vi "Old Files Handler.vi"(8 "Error In":errorcluster, 11 "TDMS Log":refnum<class "TDMS Logger.lvclass">) -> (0 "Error Out":errorcluster, 3 "TDMS Log":refnum<class "TDMS Logger.lvclass">)   [LabVIEW 2015, in "TDMS Logger.lvlib" / "TDMS Logger.lvclass"]
uses:
  TDMS Logger.lvclass
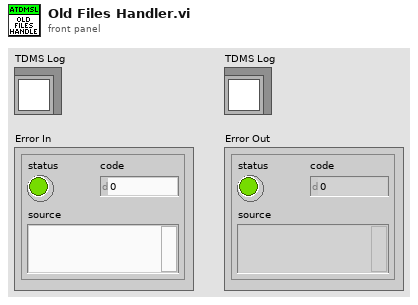
[diagram p1: front panel]
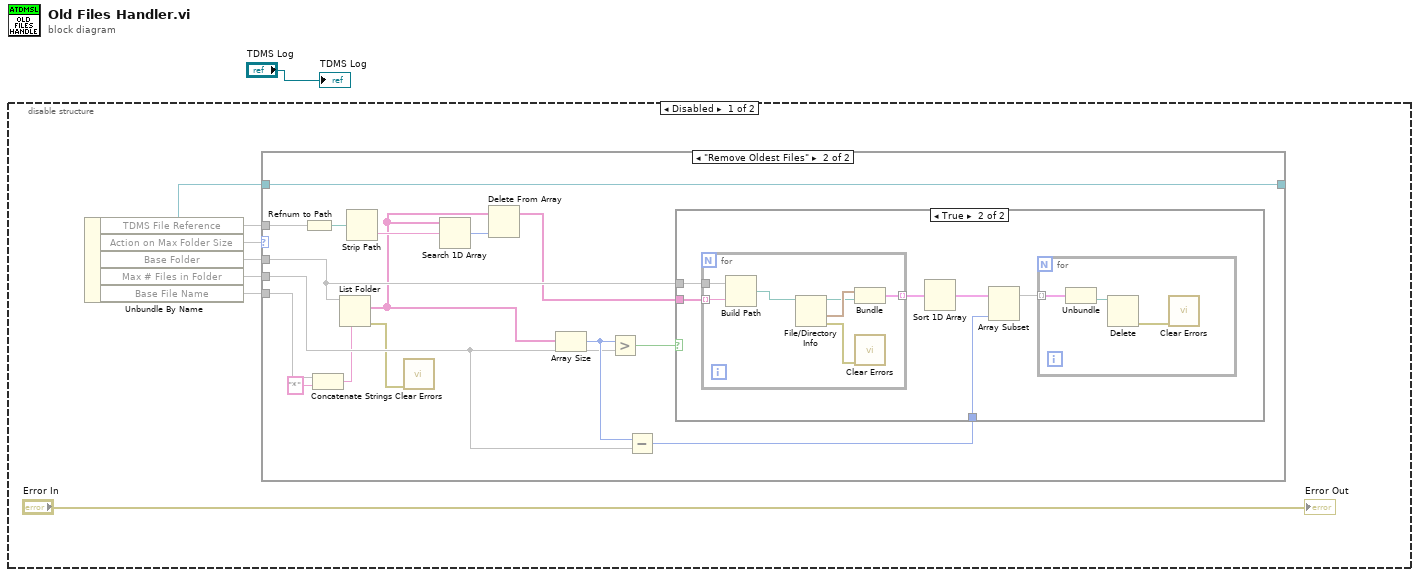
[diagram p0: block diagram]
diagram:
  n1 = disable-structure shown="Disabled" {
    frame Disabled {
      n2 = Unbundle By Name() -> (w8:refnum<class "TDMS Logger.lvclass">, "TDMS File Reference"=w4, "Action on Max Folder Size"=w6, "Base Folder"=w5, "Max # Files in Folder"=w7, "Base File Name"=w2)
      n3 = case shown="\"Remove Oldest Files\"" w6 {
        tunnel: w5 -> [_ w24]
        tunnel: w7 -> [_ w22]
        tunnel: w8 -> [w10 w25]
        tunnel: [w10 w25] -> w9
        tunnel: w4 -> [_ w20]
        tunnel: w2 -> [_ w16]
        frame "Do Nothing", Default {
        }
        frame "Remove Oldest Files" {
          n4 = Refnum to Path(1:w20) -> (0:w19:path)
          n5 = Concatenate Strings(w16, "*" ("string")) -> (w15:string)
          n6 = List Folder(path=w24, pattern=w15) -> (filenames=w11:string[], error out=w13:errorcluster)  [unwired: 2 in, 2 out]
          n7 = Strip Path(path=w19) -> (name=w18:string)  [unwired: 1 out]
          n8 = call <vilib>:"Clear Errors.vi"("error in (no error)"=w13) -> ()  [unwired: 5 in, 2 out]
          n9 = Search 1D Array(1D array=w11, element=w18) -> (index of element=w17:i32)  [unwired: 1 in]
          n10 = Delete From Array(array=w11, index=w17) -> (array with subset deleted=w12:string[])  [unwired: 1 in, 1 out]
          n11 = Array Size(array=w11) -> (size(s)=w23:i32)
          n12 = Greater?(x=w23, y=w22) -> (0:w26:bool)
          n13 = Subtract(x=w23, y=w22) -> (x-y=w21:i32)
          n14 = case shown="True" w26 {
            tunnel: w12 -> [_ w32]
            tunnel: w24 -> [_ w28]
            tunnel: w21 -> [_ w27]
            frame False {
            }
            frame True {
              n15 = for {
                tunnel: w32 -> [w39] mode=indexing
                tunnel: [w41] -> w31 mode=indexing
                tunnel: w28 -> [w38]
                n16 = Build Path(base path=w38, name or relative path=w39) -> (appended path=w37:path)
                n17 = File/Directory Info(path=w37) -> (path out=w40:path, last mod=w42:timestamp, error out=w36:errorcluster)  [unwired: 1 in, 4 out]
                n18 = Bundle("last mod"=w42, "path out"=w40) -> (w41:cluster{"last mod":timestamp, "path out":path})  [unwired: 1 in]
                n19 = call <vilib>:"Clear Errors.vi"("error in (no error)"=w36) -> ()  [unwired: 5 in, 2 out]
              }
              n20 = Sort 1D Array(array=w31) -> (sorted array=w29:cluster{"last mod":timestamp, "path out":path}[])
              n21 = Array Subset(array=w29, length=w27) -> (w30:cluster{"last mod":timestamp, "path out":path}[])  [unwired: 1 in]
              n22 = for {
                tunnel: w30 -> [w35] mode=indexing
                n23 = Unbundle(w35) -> ("path out"=w34:path)  [unwired: 1 out]
                n24 = Delete(path (use dialog)=w34) -> (error out=w33:errorcluster)  [unwired: 4 in, 2 out]
                n25 = call <vilib>:"Clear Errors.vi"("error in (no error)"=w33) -> ()  [unwired: 5 in, 2 out]
              }
            }
          }
        }
      }
      "Error Out" <- "Error In"
    }
    frame Enabled {
    }
  }
  "TDMS Log" <- "TDMS Log"
